vi "Search Enum Values.vi"(9 "Types":string[](array[string]), 10 "EnumVals":i32[](array[numeric]), 11 "String":string) -> (3 "Array out":i32[][](array[numeric]))   [LabVIEW 2020, in "Camera.lvlib"]
uses:
  Camera.lvlib
  34f12509-99c0-4568-8f7f-874d08d4582e.vi
  d3327ed6-3940-4f65-8614-4daedb81b65a.vi
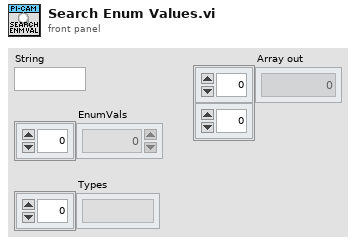
[diagram p1: front panel]
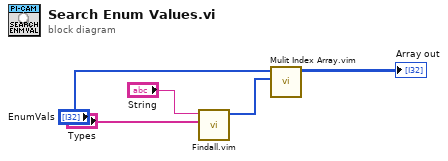
[diagram p0: block diagram]
diagram:
  n1 = call "Findall.vim"("Array"="Types", "String"="String") -> ("Array"=w4:i32[])  [unwired: 9 in]
  n2 = call "Mulit Index Array.vim"("Index Array"=w4, "Array"="EnumVals") -> ("Array out"=→"Array out":i32[][])  [unwired: 9 in]
